vi "IST.vi"(6 "lambda":dbl, 7 "Input":T1, 8 "KK":i32[][](array[numeric]), 9 "Y":dbl[][](array[numeric]), 10 "H":dbl[](array[numeric]), 11 "G":dbl[](array[numeric])) -> (2 "W":dbl[][](array[numeric]), 3 "output":T1)   [LabVIEW 2016]
uses:
  <vilib>/imath/engines/lvmath2/RunTimeEngine/IndexRead/NIMS M($,R2).vi
  <instcachedir>/0/NIMS M($,R2)_D9380E19261A4ADFB2D364AF6959C6EF.lvgen/NIMS M($,R2)_D9380E19261A4ADFB2D364AF6959C6EF_001.vi
  <vilib>/imath/engines/lvmath2/RunTimeEngine/RowToken/NIMS_RowToken_M_M.vi
  <instcachedir>/0/NIMS_RowToken_M_M_968CDE3545E74ACDAEA4B48DE01EEECA.lvgen/NIMS_RowToken_M_M_968CDE3545E74ACDAEA4B48DE01EEECA_004.vi
  <vilib>/imath/engines/lvmath2/RunTimeEngine/ErrorHandling/NIMS_Create Error From Enums.vi
  <vilib>/imath/engines/lvmath2/RunTimeEngine/BuiltInFunctions/size/NIMS_I32=size(GM,I32).vi
  <instcachedir>/0/NIMS_I32=size(GM,I32)_122058B1B3294FAEA5DC209B92B394E4.lvgen/NIMS_I32=size(GM,I32)_122058B1B3294FAEA5DC209B92B394E4_004.vi
  <vilib>/imathl/engines/lvmath/Functions/Error Handling/Create Error.vi
  <vilib>/imath/engines/lvmath2/RunTimeEngine/IndexRead/NIMS V(S).vi
  <instcachedir>/0/NIMS V(S)_0488751826AF41519A22953C041130DC.lvgen/NIMS V(S)_0488751826AF41519A22953C041130DC_000.vi
  <vilib>/imath/engines/lvmath2/RunTimeEngine/ArithmeticOperatorToken/NIMS_ArithmeticOperator_plus.vi
  <instcachedir>/0/NIMS_ArithmeticOperator_plus_0120E0498A0F4B4B9BDCAC2554767A4E.lvgen/NIMS_ArithmeticOperator_plus_0120E0498A0F4B4B9BDCAC2554767A4E_003.vi
  <vilib>/imath/engines/lvmath2/RunTimeEngine/IndexReplace/NIMS M($,R3)=M.vi
  <instcachedir>/0/NIMS M($,R3)=M_CE355598DBF149D1A5C042A13924C31E.lvgen/NIMS M($,R3)=M_CE355598DBF149D1A5C042A13924C31E_000.vi
  <vilib>/imath/engines/lvmath2/RunTimeEngine/BuiltInFunctions/size/NIMS_I32Row=size(GM).vi
  <instcachedir>/0/NIMS_I32Row=size(GM)_10ACDCB9F1F84A7E9F42C91D87611FB5.lvgen/NIMS_I32Row=size(GM)_10ACDCB9F1F84A7E9F42C91D87611FB5_001.vi
  <vilib>/imath/engines/lvmath2/RunTimeEngine/BuiltInFunctions/zeros/NIMS_M=zeros(I32V).vi
  <vilib>/imath/engines/lvmath2/RunTimeEngine/IndexRead/NIMS M(M).vi
  <instcachedir>/0/NIMS M(M)_EB00EBD471DD47B0915ED9997EB5A993.lvgen/NIMS M(M)_EB00EBD471DD47B0915ED9997EB5A993_004.vi
  <vilib>/imath/engines/lvmath2/RunTimeEngine/IndexReplace/NIMS M(M)=M.vi
  <instcachedir>/0/NIMS M(M)=M_D07272DCF1984374AF2B42254FCB82DF.lvgen/NIMS M(M)=M_D07272DCF1984374AF2B42254FCB82DF_003.vi
  <vilib>/imath/engines/lvmath2/RunTimeEngine/ArithmeticOperatorToken/NIMS_ArithmeticOperator_minus.vi
  <instcachedir>/0/NIMS_ArithmeticOperator_minus_E3B65B1D26A44BB184AFDC5B3F458E3D.lvgen/NIMS_ArithmeticOperator_minus_E3B65B1D26A44BB184AFDC5B3F458E3D_002.vi
  <vilib>/imath/engines/lvmath2/RunTimeEngine/IndexRead/NIMS M($,R3).vi
  <instcachedir>/0/NIMS M($,R3)_AF567468BD8F49DCA9979B31CBFFB5D3.lvgen/NIMS M($,R3)_AF567468BD8F49DCA9979B31CBFFB5D3_000.vi
  <vilib>/imath/engines/lvmath2/RunTimeEngine/BuiltInFunctions/abs/NIMS_abs(signed).vi
  <instcachedir>/0/NIMS_abs(signed)_C4FCB8E6058B49B797C7C8D53CA5F6EC.lvgen/NIMS_abs(signed)_C4FCB8E6058B49B797C7C8D53CA5F6EC_005.vi
  <vilib>/imath/engines/lvmath2/RunTimeEngine/VariableToken/Support/NIMS_Matrix Boolean Index to I32 Index.vi
  <vilib>/imath/engines/lvmath2/RunTimeEngine/IndexReplace/NIMS M(V)=S.vi
  <instcachedir>/0/NIMS M(V)=S_F2304187E1344F60ABCBE5C5CC0920F9.lvgen/NIMS M(V)=S_F2304187E1344F60ABCBE5C5CC0920F9_000.vi
  <vilib>/imath/engines/lvmath2/RunTimeEngine/IndexRead/NIMS M(V).vi
  <instcachedir>/0/NIMS M(V)_948FAC22C1C943948B75DA6190348614.lvgen/NIMS M(V)_948FAC22C1C943948B75DA6190348614_005.vi
  <vilib>/imath/engines/lvmath2/RunTimeEngine/IndexReplace/NIMS M(V)=M.vi
  <instcachedir>/0/NIMS M(V)=M_8AFA88AF31474F88A49F1280331F2300.lvgen/NIMS M(V)=M_8AFA88AF31474F88A49F1280331F2300_003.vi
  <vilib>/imath/engines/lvmath2/RunTimeEngine/NodeEndStatement/NIMS_NodeEndStatement_Output.vi
  <instcachedir>/0/NIMS_NodeEndStatement_Output_53EC0D466D134D7ABD903AC30B43404B.lvgen/NIMS_NodeEndStatement_Output_53EC0D466D134D7ABD903AC30B43404B_002.vi
  <vilib>/imath/engines/lvmath2/RunTimeEngine/ErrorHandling/NIMS_Finalize Error.vi
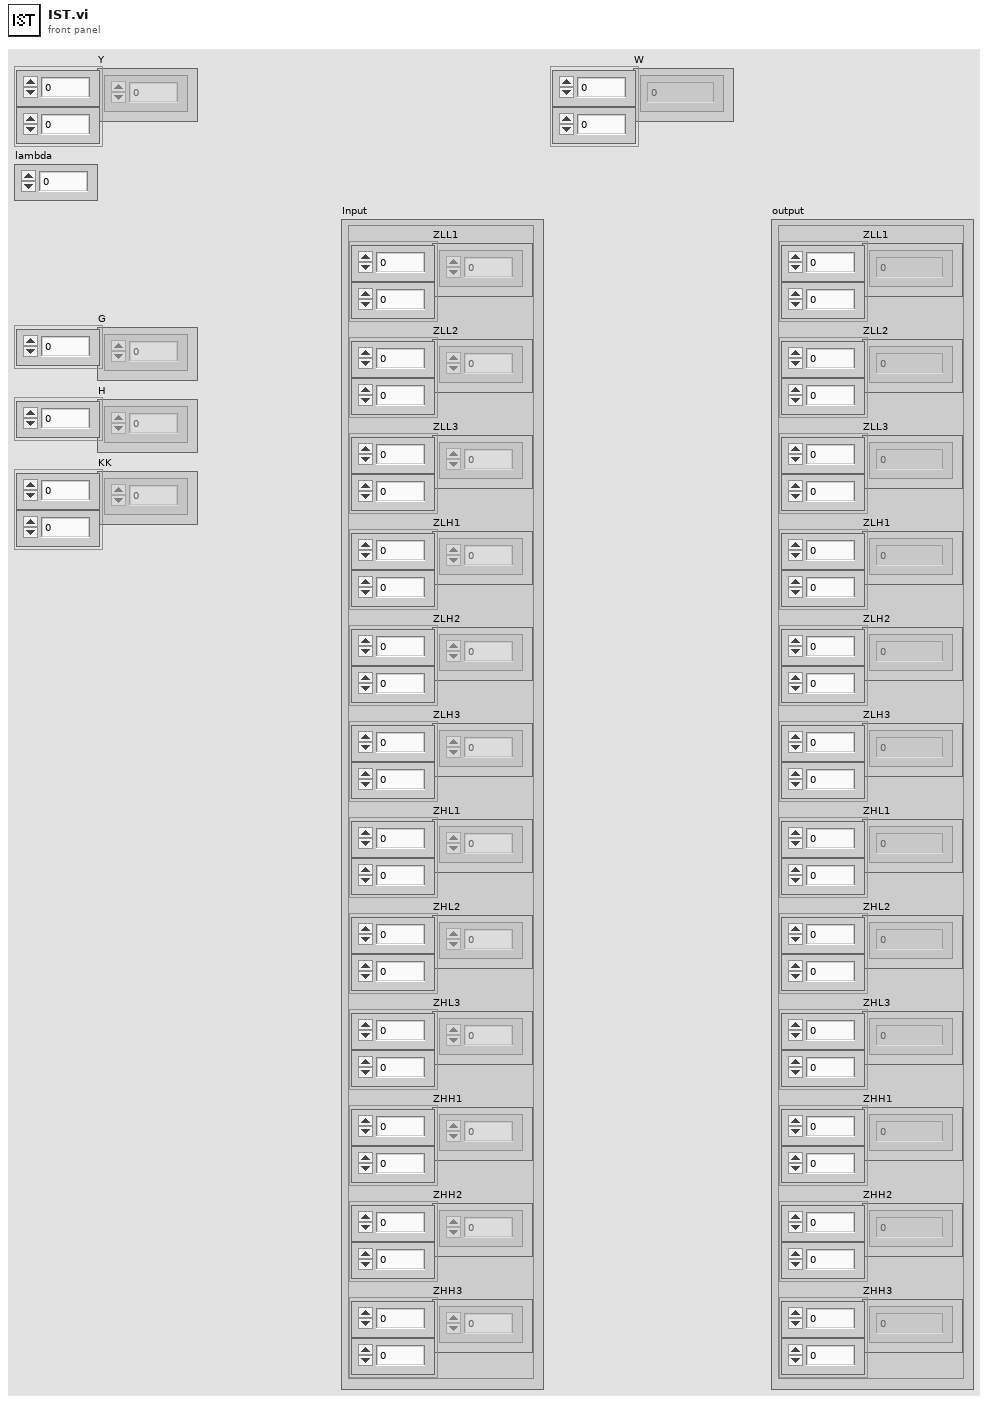
[diagram p1: front panel]
types:
  T1 = cluster{"ZLL1":dbl[][], "ZLL2":dbl[][], "ZLL3":dbl[][], "ZLH1":dbl[][], "ZLH2":dbl[][], "ZLH3":dbl[][], "ZHL1":dbl[][], "ZHL2":dbl[][], "ZHL3":dbl[][], "ZHH1":dbl[][], "ZHH2":dbl[][], "ZHH3":dbl[][]}
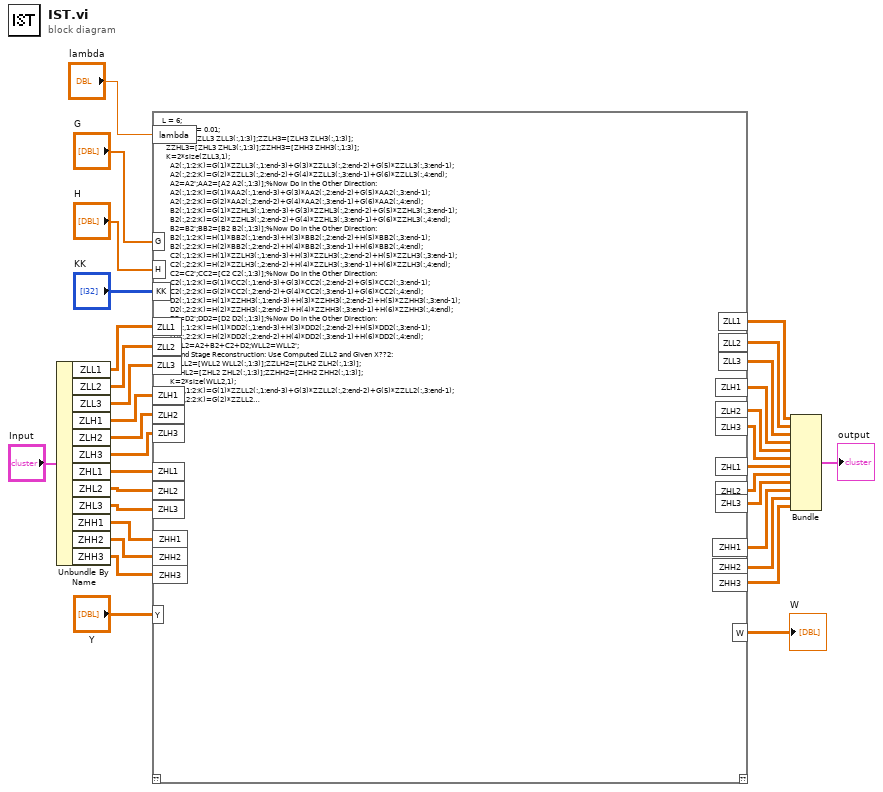
[diagram p0: block diagram]
diagram:
  n1 = Unbundle By Name("Input") -> ("ZLL1"=w28:dbl[][], "ZLL2"=w27:dbl[][], "ZLL3"=w26:dbl[][], "ZLH1"=w25:dbl[][], "ZLH2"=w24:dbl[][], "ZLH3"=w23:dbl[][], "ZHL1"=w22:dbl[][], "ZHL2"=w21:dbl[][], "ZHL3"=w20:dbl[][], "ZHH1"=w19:dbl[][], "ZHH2"=w18:dbl[][], "ZHH3"=w17:dbl[][])
  n2 = mathscript code="L = 6;\n%lambda = 0.01;\n  ZZLL3=[ZLL3 ZLL3(:,1:3)];ZZLH3=[ZLH3 ZLH3(:,1:3)];\n  ZZHL3=[ZHL3 ZHL3(:,1:3)];ZZHH3=[ZHH3 ZHH3(:,1:3)];\n  K=2*size(ZLL3,1);\n    A2(:,1:2:K)=G(1)*ZZLL3(:,1:end-3)+G(3)*ZZLL3(:,2:end-2)+G(5)*ZZLL3(:,3:end-1);\n    A2(:,2:2:K)=G(2)*ZZLL3(:,2:end-2)+G(4)*ZZLL3(:,3:end-1)+G(6)*ZZLL3(:,4:end);\n    A2=A2';AA2=[A2 A2(:,1:3)];%Now Do in the Other Direction:\n    A2(:,1:2:K)=G(1)*AA2(:,1:end-3)+G(3)*AA2(:,2:end-2)+G(5)*AA2(:,3:end-1);\n    A2(:,2:2:K)=G(2)*AA2(:,2:end-2)+G(4)*AA2(:,3:end-1)+G(6)*AA2(:,4:end);\n    B2(:,1:2:K)=G(1)*ZZHL3(:,1:end-3)+G(3)*ZZHL3(:,2:end-2)+G(5)*ZZHL3(:,3:end-1);\n    B2(:,2:2:K)=G(2)*ZZHL3(:,2:end-2)+G(4)*ZZHL3(:,3:end-1)+G(6)*ZZHL3(:,4:end);\n    B2=B2';BB2=[B2 B2(:,1:3)];%Now Do in the Other Direction:\n    B2(:,1:2:K)=H(1)*BB2(:,1:end-3)+H(3)*BB2(:,2:end-2)+H(5)*BB2(:,3:end-1);\n    B2(:,2:2:K)=H(2)*BB2(:,2:end-2)+H(4)*BB2(:,3:end-1)+H(6)*BB2(:,4:end);\n    C2(:,1:2:K)=H(1)*ZZLH3(:,1:end-3)+H(3)*ZZLH3(:,2:end-2)+H(5)*ZZLH3(:,3:end-1);\n    C2(:,2:2:K)=H(2)*ZZLH3(:,2:end-2)+H(4)*ZZLH3(:,3:end-1)+H(6)*ZZLH3(:,4:end);\n    C2=C2';CC2=[C2 C2(:,1:3)];%Now Do in the Other Direction:\n    C2(:,1:2:K)=G(1)*CC2(:,1:end-3)+G(3)*CC2(:,2:end-2)+G(5)*CC2(:,3:end-1);\n    C2(:,2:2:K)=G(2)*CC2(:,2:end-2)+G(4)*CC2(:,3:end-1)+G(6)*CC2(:,4:end);\n    D2(:,1:2:K)=H(1)*ZZHH3(:,1:end-3)+H(3)*ZZHH3(:,2:end-2)+H(5)*ZZHH3(:,3:end-1);\n    D2(:,2:2:K)=H(2)*ZZHH3(:,2:end-2)+H(4)*ZZHH3(:,3:end-1)+H(6)*ZZHH3(:,4:end);\n    D2=D2';DD2=[D2 D2(:,1:3)];%Now Do in the Other Direction:\n    D2(:,1:2:K)=H(1)*DD2(:,1:end-3)+H(3)*DD2(:,2:end-2)+H(5)*DD2(:,3:end-1);\n    D2(:,2:2:K)=H(2)*DD2(:,2:end-2)+H(4)*DD2(:,3:end-1)+H(6)*DD2(:,4:end);\n    WLL2=A2+B2+C2+D2;WLL2=WLL2';\n    %2nd Stage Reconstruction: Use Computed ZLL2 and Given X??2:\n    ZZLL2=[WLL2 WLL2(:,1:3)];ZZLH2=[ZLH2 ZLH2(:,1:3)];\n    ZZHL2=[ZHL2 ZHL2(:,1:3)];ZZHH2=[ZHH2 ZHH2(:,1:3)];\n    K=2*size(WLL2,1);\n    A1(:,1:2:K)=G(1)*ZZLL2(:,1:end-3)+G(3)*ZZLL2(:,2:end-2)+G(5)*ZZLL2(:,3:end-1);\n    A1(:,2:2:K)=G(2)*ZZLL2(:,2:end-2)+G(4)*ZZLL2(:,3:end-1)+G(6)*ZZLL2(:,4:end);\n    A1=A1';AA1=[A1 A1(:,1:3)];%Now Do in the Other Direction:\n    A1(:,1:2:K)=G(1)*AA1(:,1:end-3)+G(3)*AA1(:,2:end-2)+G(5)*AA1(:,3:end-1);\n    A1(:,2:2:K)=G(2)*AA1(:,2:end-2)+G(4)*AA1(:,3:end-1)+G(6)*AA1(:,4:end);\n    B1(:,1:2:K)=G(1)*ZZHL2(:,1:end-3)+G(3)*ZZHL2(:,2:end-2)+G(5)*ZZHL2(:,3:end-1);\n    B1(:,2:2:K)=G(2)*ZZHL2(:,2:end-2)+G(4)*ZZHL2(:,3:end-1)+G(6)*ZZHL2(:,4:end);\n    B1=B1';BB1=[B1 B1(:,1:3)];%Now Do in the Other Direction:\n    B1(:,1:2:K)=H(1)*BB1(:,1:end-3)+H(3)*BB1(:,2:end-2)+H(5)*BB1(:,3:end-1);\n    B1(:,2:2:K)=H(2)*BB1(:,2:end-2)+H(4)*BB1(:,3:end-1)+H(6)*BB1(:,4:end);\n    C1(:,1:2:K)=H(1)*ZZLH2(:,1:end-3)+H(3)*ZZLH2(:,2:end-2)+H(5)*ZZLH2(:,3:end-1);\n    C1(:,2:2:K)=H(2)*ZZLH2(:,2:end-2)+H(4)*ZZLH2(:,3:end-1)+H(6)*ZZLH2(:,4:end);\n    C1=C1';CC1=[C1 C1(:,1:3)];%Now Do in the Other Direction:\n    C1(:,1:2:K)=G(1)*CC1(:,1:end-3)+G(3)*CC1(:,2:end-2)+G(5)*CC1(:,3:end-1);\n    C1(:,2:2:K)=G(2)*CC1(:,2:end-2)+G(4)*CC1(:,3:end-1)+G(6)*CC1(:,4:end);\n    D1(:,1:2:K)=H(1)*ZZHH2(:,1:end-3)+H(3)*ZZHH2(:,2:end-2)+H(5)*ZZHH2(:,3:end-1);\n    D1(:,2:2:K)=H(2)*ZZHH2(:,2:end-2)+H(4)*ZZHH2(:,3:end-1)+H(6)*ZZHH2(:,4:end);\n    D1=D1';DD1=[D1 D1(:,1:3)];%Now Do in the Other Direction:\n    D1(:,1:2:K)=H(1)*DD1(:,1:end-3)+H(3)*DD1(:,2:end-2)+H(5)*DD1(:,3:end-1);\n    D1(:,2:2:K)=H(2)*DD1(:,2:end-2)+H(4)*DD1(:,3:end-1)+H(6)*DD1(:,4:end);\n    WLL1=A1+B1+C1+D1;WLL1=WLL1';\n    %1st Stage Reconstruction: Use Computed ZLL1 and Given X??1:\n    ZZLL1=[WLL1 WLL1(:,1:3)];ZZLH1=[ZLH1 ZLH1(:,1:3)];\n    ZZHL1=[ZHL1 ZHL1(:,1:3)];ZZHH1=[ZHH1 ZHH1(:,1:3)];\n    K=2*size(WLL1,1);\n    A0(:,1:2:K)=G(1)*ZZLL1(:,1:end-3)+G(3)*ZZLL1(:,2:end-2)+G(5)*ZZLL1(:,3:end-1);\n    A0(:,2:2:K)=G(2)*ZZLL1(:,2:end-2)+G(4)*ZZLL1(:,3:end-1)+G(6)*ZZLL1(:,4:end);\n    A0=A0';AA0=[A0 A0(:,1:3)];%Now Do in the Other Direction:\n    A0(:,1:2:K)=G(1)*AA0(:,1:end-3)+G(3)*AA0(:,2:end-2)+G(5)*AA0(:,3:end-1);\n    A0(:,2:2:K)=G(2)*AA0(:,2:end-2)+G(4)*AA0(:,3:end-1)+G(6)*AA0(:,4:end);\n    B0(:,1:2:K)=G(1)*ZZHL1(:,1:end-3)+G(3)*ZZHL1(:,2:end-2)+G(5)*ZZHL1(:,3:end-1);\n    B0(:,2:2:K)=G(2)*ZZHL1(:,2:end-2)+G(4)*ZZHL1(:,3:end-1)+G(6)*ZZHL1(:,4:end);\n    B0=B0';BB0=[B0 B0(:,1:3)];%Now Do in the Other Direction:\n    B0(:,1:2:K)=H(1)*BB0(:,1:end-3)+H(3)*BB0(:,2:end-2)+H(5)*BB0(:,3:end-1);\n    B0(:,2:2:K)=H(2)*BB0(:,2:end-2)+H(4)*BB0(:,3:end-1)+H(6)*BB0(:,4:end);\n    C0(:,1:2:K)=H(1)*ZZLH1(:,1:end-3)+H(3)*ZZLH1(:,2:end-2)+H(5)*ZZLH1(:,3:end-1);\n    C0(:,2:2:K)=H(2)*ZZLH1(:,2:end-2)+H(4)*ZZLH1(:,3:end-1)+H(6)*ZZLH1(:,4:end);\n    C0=C0';CC0=[C0 C0(:,1:3)];%Now Do in the Other Direction:\n    C0(:,1:2:K)=G(1)*CC0(:,1:end-3)+G(3)*CC0(:,2:end-2)+G(5)*CC0(:,3:end-1);\n    C0(:,2:2:K)=G(2)*CC0(:,2:end-2)+G(4)*CC0(:,3:end-1)+G(6)*CC0(:,4:end);\n    D0(:,1:2:K)=H(1)*ZZHH1(:,1:end-3)+H(3)*ZZHH1(:,2:end-2)+H(5)*ZZHH1(:,3:end-1);\n    D0(:,2:2:K)=H(2)*ZZHH1(:,2:end-2)+H(4)*ZZHH1(:,3:end-1)+H(6)*ZZHH1(:,4:end);\n    D0=D0';DD0=[D0 D0(:,1:3)];%Now Do in the Other Direction:\n    D0(:,1:2:K)=H(1)*DD0(:,1:end-3)+H(3)*DD0(:,2:end-2)+H(5)*DD0(:,3:end-1);\n    D0(:,2:2:K)=H(2)*DD0(:,2:end-2)+H(4)*DD0(:,3:end-1)+H(6)*DD0(:,4:end);\n    WLL0=A0+B0+C0+D0;W=WLL0';\n    %End inverse wavelet transform:Z->W\nWK = zeros(size(W));\n    WK(KK)=W(KK);YWK=Y-WK;%D=F'(y-FH'z^{k}).\n    %HF'(y-FH'z^{k})=HF'(FD)=HD=H(YWK).\n    %Now wavelet transform of YWK:{X???}\n    %1st Stage D3 Daubechies Wavelet Transform:\n    XXLL0=[YWK(:,end-L+2:end) YWK];%Cyclic Pre-padding\n    XLL1=G(1)*XXLL0(:,L:2:end-1)+G(2)*XXLL0(:,L-1:2:end-2)+G(3)*XXLL0(:,L-2:2:end-3);\n    XLL1=XLL1+G(4)*XXLL0(:,L-3:2:end-4)+G(5)*XXLL0(:,L-4:2:end-5)+G(6)*XXLL0(:,L-5:2:end-6);\n    XHH1=H(1)*XXLL0(:,L:2:end-1)+H(2)*XXLL0(:,L-1:2:end-2)+H(3)*XXLL0(:,L-2:2:end-3);\n    XHH1=XHH1+H(4)*XXLL0(:,L-3:2:end-4)+H(5)*XXLL0(:,L-4:2:end-5)+H(6)*XXLL0(:,L-5:2:end-6);\n    XLL1=XLL1';XHH1=XHH1';%Now Do in the Other Direction:\n    XXLL1=[XLL1(:,end-L+2:end) XLL1];XXHH1=[XHH1(:,end-L+2:end) XHH1];%Cyclic Pre-padding\n    XLL1=G(1)*XXLL1(:,L:2:end-1)+G(2)*XXLL1(:,L-1:2:end-2)+G(3)*XXLL1(:,L-2:2:end-3);\n    XLL1=XLL1+G(4)*XXLL1(:,L-3:2:end-4)+G(5)*XXLL1(:,L-4:2:end-5)+G(6)*XXLL1(:,L-5:2:end-6);\n    XHH1=H(1)*XXHH1(:,L:2:end-1)+H(2)*XXHH1(:,L-1:2:end-2)+H(3)*XXHH1(:,L-2:2:end-3);\n    XHH1=XHH1+H(4)*XXHH1(:,L-3:2:end-4)+H(5)*XXHH1(:,L-4:2:end-5)+H(6)*XXHH1(:,L-5:2:end-6);\n    XHL1=H(1)*XXLL1(:,L:2:end-1)+H(2)*XXLL1(:,L-1:2:end-2)+H(3)*XXLL1(:,L-2:2:end-3);\n    XHL1=XHL1+H(4)*XXLL1(:,L-3:2:end-4)+H(5)*XXLL1(:,L-4:2:end-5)+H(6)*XXLL1(:,L-5:2:end-6);\n    XLH1=G(1)*XXHH1(:,L:2:end-1)+G(2)*XXHH1(:,L-1:2:end-2)+G(3)*XXHH1(:,L-2:2:end-3);\n    XLH1=XLH1+G(4)*XXHH1(:,L-3:2:end-4)+G(5)*XXHH1(:,L-4:2:end-5)+G(6)*XXHH1(:,L-5:2:end-6);\n    XLL1=XLL1';XHH1=XHH1';XHL1=XHL1';XLH1=XLH1';\n    %2nd Stage D3 Daubechies Wavelet Transform:\n    XXLL1=[XLL1(:,end-L+2:end) XLL1];%Cyclic Pre-padding\n    XLL2=G(1)*XXLL1(:,L:2:end-1)+G(2)*XXLL1(:,L-1:2:end-2)+G(3)*XXLL1(:,L-2:2:end-3);\n    XLL2=XLL2+G(4)*XXLL1(:,L-3:2:end-4)+G(5)*XXLL1(:,L-4:2:end-5)+G(6)*XXLL1(:,L-5:2:end-6);\n    XHH2=H(1)*XXLL1(:,L:2:end-1)+H(2)*XXLL1(:,L-1:2:end-2)+H(3)*XXLL1(:,L-2:2:end-3);\n    XHH2=XHH2+H(4)*XXLL1(:,L-3:2:end-4)+H(5)*XXLL1(:,L-4:2:end-5)+H(6)*XXLL1(:,L-5:2:end-6);\n    XLL2=XLL2';XHH2=XHH2';%Now Do in the Other Direction:\n    XXLL2=[XLL2(:,end-L+2:end) XLL2];XXHH2=[XHH2(:,end-L+2:end) XHH2];%Cyclic Pre-padding\n    XLL2=G(1)*XXLL2(:,L:2:end-1)+G(2)*XXLL2(:,L-1:2:end-2)+G(3)*XXLL2(:,L-2:2:end-3);\n    XLL2=XLL2+G(4)*XXLL2(:,L-3:2:end-4)+G(5)*XXLL2(:,L-4:2:end-5)+G(6)*XXLL2(:,L-5:2:end-6);\n    XHH2=H(1)*XXHH2(:,L:2:end-1)+H(2)*XXHH2(:,L-1:2:end-2)+H(3)*XXHH2(:,L-2:2:end-3);\n    XHH2=XHH2+H(4)*XXHH2(:,L-3:2:end-4)+H(5)*XXHH2(:,L-4:2:end-5)+H(6)*XXHH2(:,L-5:2:end-6);\n    XHL2=H(1)*XXLL2(:,L:2:end-1)+H(2)*XXLL2(:,L-1:2:end-2)+H(3)*XXLL2(:,L-2:2:end-3);\n    XHL2=XHL2+H(4)*XXLL2(:,L-3:2:end-4)+H(5)*XXLL2(:,L-4:2:end-5)+H(6)*XXLL2(:,L-5:2:end-6);\n    XLH2=G(1)*XXHH2(:,L:2:end-1)+G(2)*XXHH2(:,L-1:2:end-2)+G(3)*XXHH2(:,L-2:2:end-3);\n    XLH2=XLH2+G(4)*XXHH2(:,L-3:2:end-4)+G(5)*XXHH2(:,L-4:2:end-5)+G(6)*XXHH2(:,L-5:2:end-6);\n    XLL2=XLL2';XHH2=XHH2';XHL2=XHL2';XLH2=XLH2';\n    %3rd Stage D3 Daubechies Wavelet Transform:\n    XXLL2=[XLL2(:,end-L+2:end) XLL2];%Cyclic Pre-padding\n    XLL3=G(1)*XXLL2(:,L:2:end-1)+G(2)*XXLL2(:,L-1:2:end-2)+G(3)*XXLL2(:,L-2:2:end-3);\n    XLL3=XLL3+G(4)*XXLL2(:,L-3:2:end-4)+G(5)*XXLL2(:,L-4:2:end-5)+G(6)*XXLL2(:,L-5:2:end-6);\n    XHH3=H(1)*XXLL2(:,L:2:end-1)+H(2)*XXLL2(:,L-1:2:end-2)+H(3)*XXLL2(:,L-2:2:end-3);\n    XHH3=XHH3+H(4)*XXLL2(:,L-3:2:end-4)+H(5)*XXLL2(:,L-4:2:end-5)+H(6)*XXLL2(:,L-5:2:end-6);\n    XLL3=XLL3';XHH3=XHH3';%Now Do in the Other Direction:\n    XXLL3=[XLL3(:,end-L+2:end) XLL3];XXHH3=[XHH3(:,end-L+2:end) XHH3];%Cyclic Pre-padding\n    XLL3=G(1)*XXLL3(:,L:2:end-1)+G(2)*XXLL3(:,L-1:2:end-2)+G(3)*XXLL3(:,L-2:2:end-3);\n    XLL3=XLL3+G(4)*XXLL3(:,L-3:2:end-4)+G(5)*XXLL3(:,L-4:2:end-5)+G(6)*XXLL3(:,L-5:2:end-6);\n    XHH3=H(1)*XXHH3(:,L:2:end-1)+H(2)*XXHH3(:,L-1:2:end-2)+H(3)*XXHH3(:,L-2:2:end-3);\n    XHH3=XHH3+H(4)*XXHH3(:,L-3:2:end-4)+H(5)*XXHH3(:,L-4:2:end-5)+H(6)*XXHH3(:,L-5:2:end-6);\n    XHL3=H(1)*XXLL3(:,L:2:end-1)+H(2)*XXLL3(:,L-1:2:end-2)+H(3)*XXLL3(:,L-2:2:end-3);\n    XHL3=XHL3+H(4)*XXLL3(:,L-3:2:end-4)+H(5)*XXLL3(:,L-4:2:end-5)+H(6)*XXLL3(:,L-5:2:end-6);\n    XLH3=G(1)*XXHH3(:,L:2:end-1)+G(2)*XXHH3(:,L-1:2:end-2)+G(3)*XXHH3(:,L-2:2:end-3);\n    XLH3=XLH3+G(4)*XXHH3(:,L-3:2:end-4)+G(5)*XXHH3(:,L-4:2:end-5)+G(6)*XXHH3(:,L-5:2:end-6);\n    XLL3=XLL3';XHH3=XHH3';XHL3=XHL3';XLH3=XLH3';\n    %End wavelet transform of DYWK->X???.\n    %z^{k+1}=z^{k}+HF'(y-FH'z^{k}):Now add z^{k}:\n    ZLH1=ZLH1+XLH1;ZHL1=ZHL1+XHL1;ZHH1=ZHH1+XHH1;\n    ZLH2=ZLH2+XLH2;ZHL2=ZHL2+XHL2;ZHH2=ZHH2+XHH2;\n    ZLH3=ZLH3+XLH3;ZHL3=ZHL3+XHL3;ZHH3=ZHH3+XHH3;\n    ZLL3=ZLL3+XLL3;%Only use finest-scale average.\n    %First, threshold small values to 0.\n    ZLH1(abs(ZLH1)<lambda)=0;ZHL1(abs(ZHL1)<lambda)=0;\n    ZLH2(abs(ZLH2)<lambda)=0;ZHL2(abs(ZHL2)<lambda)=0;\n    ZLH3(abs(ZLH3)<lambda)=0;ZHL3(abs(ZHL3)<lambda)=0;\n    ZHH1(abs(ZHH1)<lambda)=0;ZHH2(abs(ZHH2)<lambda)=0;\n    ZHH3(abs(ZHH3)<lambda)=0;ZLL3(abs(ZLL3)<lambda)=0;\n    %Shrink non-small values of Z???:\n    ZLH1(abs(ZLH1)>lambda)=ZLH1(abs(ZLH1)>lambda)-lambda*sign(ZLH1(abs(ZLH1)>lambda));\n    ZLH2(abs(ZLH2)>lambda)=ZLH2(abs(ZLH2)>lambda)-lambda*sign(ZLH2(abs(ZLH2)>lambda));\n    ZLH3(abs(ZLH3)>lambda)=ZLH3(abs(ZLH3)>lambda)-lambda*sign(ZLH3(abs(ZLH3)>lambda));\n    ZHL1(abs(ZHL1)>lambda)=ZHL1(abs(ZHL1)>lambda)-lambda*sign(ZHL1(abs(ZHL1)>lambda));\n    ZHL2(abs(ZHL2)>lambda)=ZHL2(abs(ZHL2)>lambda)-lambda*sign(ZHL2(abs(ZHL2)>lambda));\n    ZHL3(abs(ZHL3)>lambda)=ZHL3(abs(ZHL3)>lambda)-lambda*sign(ZHL3(abs(ZHL3)>lambda));\n    ZHH1(abs(ZHH1)>lambda)=ZHH1(abs(ZHH1)>lambda)-lambda*sign(ZHH1(abs(ZHH1)>lambda));\n    ZHH2(abs(ZHH2)>lambda)=ZHH2(abs(ZHH2)>lambda)-lambda*sign(ZHH2(abs(ZHH2)>lambda));\n    ZHH3(abs(ZHH3)>lambda)=ZHH3(abs(ZHH3)>lambda)-lambda*sign(ZHH3(abs(ZHH3)>lambda));\n    ZLL3(abs(ZLL3)>lambda)=ZLL3(abs(ZLL3)>lambda)-lambda*sign(ZLL3(abs(ZLL3)>lambda));"("ZHH1"=w19, "ZHH2"=w18, "ZHH3"=w17, "ZLL1"=w28, "ZLL2"=w27, "ZLH3"=w23, "ZLL3"=w26, "ZLH1"=w25, "ZLH2"=w24, "ZHL1"=w22, "ZHL2"=w21, "ZHL3"=w20, "G"="G", "H"="H", "KK"="KK", "Y"="Y", "lambda"="lambda") -> ("ZLL2"=w15:dbl[][], "ZLL1"=w16:dbl[][], "ZLL3"=w14:dbl[][], "ZLH1"=w13:dbl[][], "ZLH2"=w12:dbl[][], "ZLH3"=w11:dbl[][], "ZHL1"=w9:dbl[][], "ZHL2"=w8:dbl[][], "ZHL3"=w7:dbl[][], "ZHH1"=w6:dbl[][], "ZHH2"=w5:dbl[][], "ZHH3"=w4:dbl[][], "W"=→"W":dbl[][])  [unwired: 1 in, 1 out]
  n3 = Bundle("ZLL1"=w16, "ZLL2"=w15, "ZLL3"=w14, "ZLH1"=w13, "ZLH2"=w12, "ZLH3"=w11, "ZHL1"=w9, "ZHL2"=w8, "ZHL3"=w7, "ZHH1"=w6, "ZHH2"=w5, "ZHH3"=w4) -> (→"output":T1)  [unwired: 1 in]
